vi "Get State String Info.vi"(8 "error in (no error)":errorcluster, 10 "StrCnst Refnum in":refnum<vi>, 11 "JKI SM in":refnum<class "JKI SM.lvclass">) -> (0 "error out":errorcluster, 1 "Frame Name":string, 2 "Structure":string, 3 "JKI SM out":refnum<class "JKI SM.lvclass">)   [LabVIEW 2013, in "JKI State Machine API.lvlib" / "JKI SM.lvclass"]
uses:
  JKI SM.lvclass
  JKI SM.lvclass/JKI SM.ctl
panel:
  out "Class Name":string
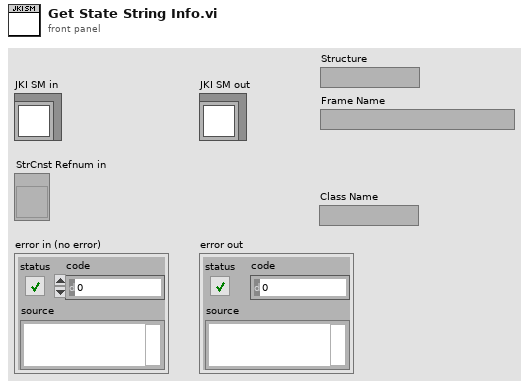
[diagram p1: front panel]
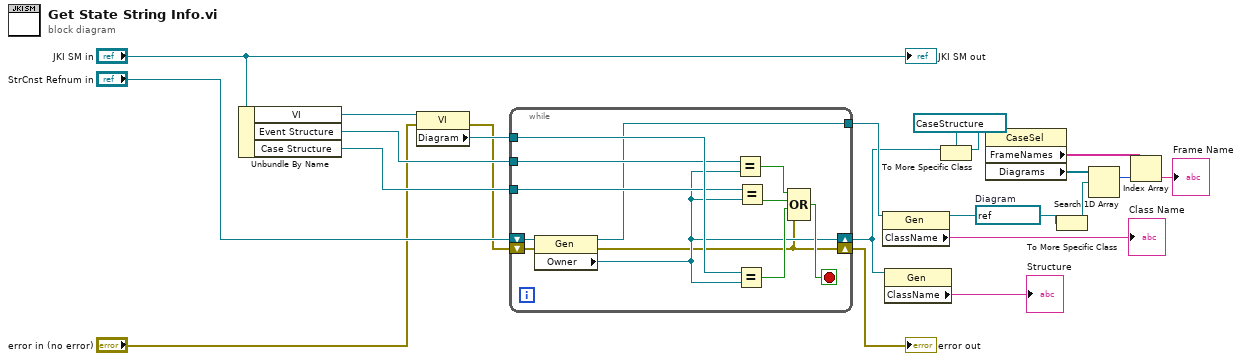
[diagram p0: block diagram]
diagram:
  w6 = refnum<vi> refnum  # Diagram
  n1 = Unbundle By Name("JKI SM in") -> ("VI"=w20:refnum<vi>, "Event Structure"=w18:refnum<vi>, "Case Structure"=w17:refnum<vi>)
  n2 = property class="VI"(reference=w20, error in="error in (no error)") -> (error out=w10:errorcluster, "Diagram"=w19:refnum<vi>)  [unwired: 1 out]
  n3 = while {
    shift-right: [w26] -> w11
    shift-left: "StrCnst Refnum in" -> [w34]
    tunnel: w19 -> [w33]
    tunnel: w18 -> [w32]
    tunnel: w17 -> [w28]
    tunnel: [w25] -> w14
    shift-right: [w23] -> w8
    shift-left: w10 -> [w24]
    stop <- w29 stop-if-true
    n4 = property class="Gen"(reference=w34, error in=w24) -> (reference out=w25:refnum<vi>, error out=w23:errorcluster, "Owner"=w26:refnum<vi>)
    n5 = Equal?(x=w32, y=w26) -> (x = y?=w31:bool)
    n6 = Equal?(x=w33, y=w26) -> (x = y?=w30:bool)
    n7 = Equal?(x=w28, y=w26) -> (x = y?=w27:bool)
    n8 = Compound Arithmetic op=OR(w31, w27, w30, w23) -> (w29:bool)
  }
  "error out" <- w8
  n9 = property class="Gen"(reference=w14) -> (reference out=w5:refnum<vi>, "ClassName"=→"Class Name":string)  [unwired: 1 in, 1 out]
  n10 = property class="Gen"(reference=w11) -> ("ClassName"=→"Structure":string)  [unwired: 1 in, 2 out]
  n11 = To More Specific Class(target class=refnum<vi> refnum ("Part References.Case Structure"), reference=w11) -> (specific class reference=w12:refnum<vi>)  [unwired: 1 in, 1 out]
  n12 = property class="CaseSel"(reference=w12) -> ("FrameNames"=w2:string[], "Diagrams"=w7:refnum<vi>[])  [unwired: 1 in, 2 out]
  n13 = To More Specific Class(target class=w6, reference=w5) -> (specific class reference=w4:refnum<vi>)  [unwired: 1 in, 1 out]
  n14 = Search 1D Array(1D array=w7, element=w4) -> (index of element=w3:i32)  [unwired: 1 in]
  n15 = Index Array(array=w2, index=w3) -> (element=→"Frame Name":string)
  "JKI SM out" <- "JKI SM in"
